vi "TEST rect and polar.vi"() -> ()   [LabVIEW 2023]
panel:
  out "output":T1(array[cluster]) {"X" format="%#.3f"; "Y" format="%#.3f"; "Magnitude" format="%#.3f"; "angle (deg)" format="%#.3f"}
  in  "input":T2(array[cluster])
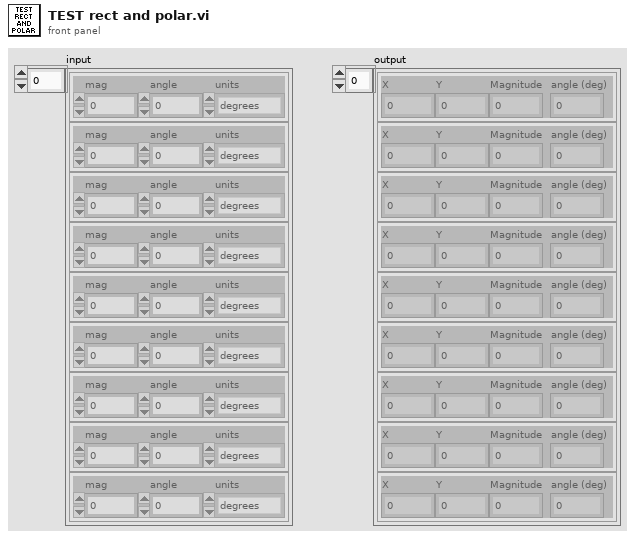
[diagram p1: front panel]
types:
  T1 = cluster{"X":dbl, "Y":dbl, "Magnitude":dbl, "angle (deg)":dbl}[]
  T2 = cluster{"mag":dbl, "angle":dbl, "units":enum16{"degrees", "radians"}}[]
  T3 = cluster{"X":dbl, "Y":dbl, "Magnitude":dbl, "angle (deg)":dbl}
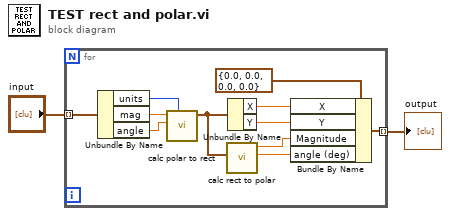
[diagram p0: block diagram]
diagram:
  n1 = for {
    tunnel: "input" -> [w13] mode=indexing
    tunnel: [w3] -> w1 mode=indexing
    n2 = Unbundle By Name(w13) -> ("units"=w10:enum16{"degrees", "radians"}, "mag"=w12:dbl, "angle"=w11:dbl)
    n3 = call "calc polar to rect.vi"("units"=w10, "angle"=w11, "mag"=w12) -> ("XY"=w8:cluster{"X":dbl, "Y":dbl})  [unwired: 8 in]
    n4 = call "calc rect to polar.vi"("XY"=w8) -> ("angle (deg)"=w4:dbl, "Magnitude"=w5:dbl)  [unwired: 8 in, 1 out]
    n5 = Unbundle By Name(w8) -> ("X"=w7:dbl, "Y"=w6:dbl)
    n6 = Bundle By Name(cluster=T3 {"X"=0.0, "Y"=0.0, "Magnitude"=0.0, "angle (deg)"=0.0} ("XY"), "X"=w7, "Y"=w6, "Magnitude"=w5, "angle (deg)"=w4) -> (w3:T3)
  }
  "output" <- w1
